vi "Task.vi"() -> (0 "error out":errorcluster)   [LabVIEW 2024]
uses:
  Devices/PCAN/PCAN.lvclass
  ConfigFromJSON/Config from JSON.lvclass
  DBCCommunication/DBC Communication.lvclass
  Devices/HSU MCU V2/HSU MCU V2.lvclass
  Instrument Factory/Instrument Factory.lvclass
  Devices/PCAN/Config Hardcoded/Config Hardcoded.lvclass
  Interfaces/IConfigure/IConfigure.lvclass
  Config from XML/Config from XML.lvclass
panel:
  in  "CAN Adapter Config":T1(ring)
  in  "CAN Adapter":enum16{"PCAN", "X-NET"}(ring)
  out "Temp Winding":dbl
  in  "Stop":bool
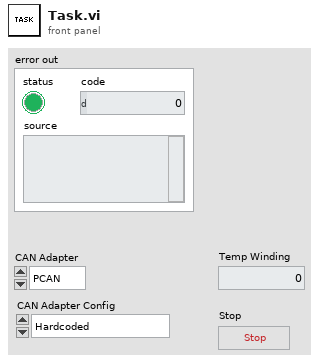
[diagram p1: front panel]
types:
  T1 = enum16{"Hardcoded", "Tests\\PCANconfig.xml", "Tests\\PCANconfig.json"}
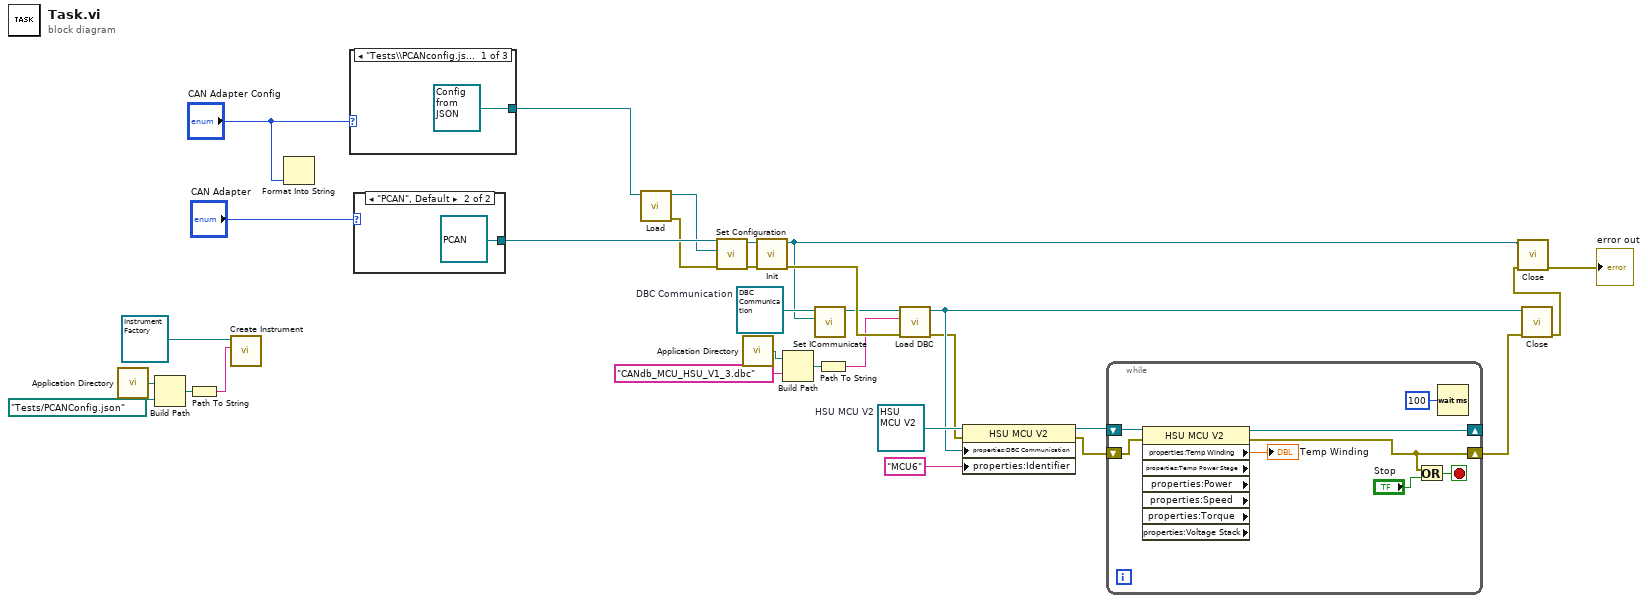
[diagram p0: block diagram]
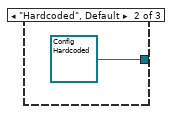
[diagram p3: hidden frame]
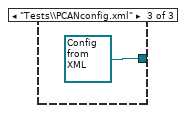
[diagram p4: hidden frame]
diagram:
  w16 = refnum<class "HSU MCU V2.lvclass"> refnum  # HSU MCU V2
  w25 = refnum<class "DBC Communication.lvclass"> refnum  # DBC Communication
  n1 = call <vilib>:"Application Directory.vi"() -> ("Application Directory"=w4:path)
  n2 = Build Path(base path=w4, name or relative path=path "Tests/PCANConfig.json") -> (appended path=w3:path)
  n3 = Path To String(path=w3) -> (string=w1:string)
  n4 = call "Create Instrument.vi"("Source"=w1, "Instrument Factory in"=refnum<class "Instrument Factory.lvclass"> refnum ("Instrument Factory.lvclass")) -> ()  [unwired: 8 in, 2 out]
  n5 = Format Into String("CAN Adapter Config") -> (resulting string=w7:string)  [unwired: 3 in, 1 out]
  n6 = case shown="\"Tests\\\\PCANconfig.json\"" "CAN Adapter Config" {
    tunnel: [refnum<class "Config from JSON.lvclass"> refnum ("Config from JSON.lvclass") refnum<class "Config Hardcoded.lvclass"> refnum ("PCAN.lvlib:Config Hardcoded.lvclass") refnum<class "Config from XML.lvclass"> refnum ("Config from XML.lvclass")] -> w29
    frame "Tests\\PCANconfig.json" {
    }
    frame "Hardcoded", Default {
    }
    frame "Tests\\PCANconfig.xml" {
    }
  }
  n7 = case shown="\"PCAN\", Default" "CAN Adapter" {
    tunnel: [_ refnum<class "PCAN.lvclass"> refnum ("PCAN CAN Adapter")] -> w31
    frame "X-NET" {
    }
    frame "PCAN", Default {
    }
  }
  n8 = call-dynamic "Load.vi"("IConfigure in"=w29) -> ("error out"=w27:errorcluster, "IConfigure out"=w26:refnum<class "IConfigure.lvclass">, "Source"=w17:string)  [unwired: 8 in]
  n9 = call-dynamic "Set Configuration.vi"("IConfigure"=w26, "Copy of PCAN in"=w31) -> ("Copy of PCAN out"=w30:refnum<class "PCAN.lvclass">)  [unwired: 9 in]
  n10 = call <vilib>:"Application Directory.vi"() -> ("Application Directory"=w23:path)
  n11 = call-dynamic "Init.vi"("error in"=w27, "PCAN in"=w30) -> ("error out"=w24:errorcluster, "PCAN out"=w18:refnum<class "PCAN.lvclass">)  [unwired: 8 in]
  n12 = Build Path(base path=w23, name or relative path="CANdb_MCU_HSU_V1_3.dbc" ("Source")) -> (appended path=w21:path)
  n13 = call "Set ICommunicate.vi"("ICommunicate"=w18, "DBCCommunication in"=w25) -> ("DBCCommunication out"=w19:refnum<class "DBC Communication.lvclass">)  [unwired: 9 in]
  n14 = Path To String(path=w21) -> (string=w20:string)
  n15 = call "Load DBC.vi"("error in"=w24, "DBC File"=w20, "DBCCommunication in"=w19) -> ("error out"=w11:errorcluster, "DBCCommunication out"=w12:refnum<class "DBC Communication.lvclass">)  [unwired: 7 in]
  n16 = property class="HSU MCU V2"(reference=w16, error in=w11, "properties:DBC Communication"=w12, "properties:Identifier"="MCU6" ("Instrument Identifier")) -> (reference out=w15:refnum<class "HSU MCU V2.lvclass">, error out=w14:errorcluster)
  n17 = while {
    shift-right: [w36] -> w10
    shift-left: w14 -> [w38]
    shift-right: [w39] -> _
    shift-left: w15 -> [w40]
    stop <- w42 stop-if-true
    n18 = property class="HSU MCU V2" props=["properties:Temp Winding", "properties:Temp Power Stage", "properties:Power", "properties:Speed ", "properties:Torque", "properties:Voltage Stack"](reference=w40, error in=w38) -> (reference out=w39:refnum<class "HSU MCU V2.lvclass">, error out=w36:errorcluster, "properties:Temp Winding"=→"Temp Winding":dbl)  [unwired: 5 out]
    n19 = Or(x=w36, y="Stop") -> (x .or. y?=w42:bool)
    n20 = Wait (ms)(milliseconds to wait=u32 100) -> ()  [unwired: 1 out]
  }
  n21 = call-dynamic "Close.vi"("error in"=w10, "DBC Communication in"=w12) -> ("error out"=w9:errorcluster)  [unwired: 8 in, 1 out]
  n22 = call-dynamic "Close.vi"("error in"=w9, "PCAN in"=w18) -> ("error out"=→"error out":errorcluster)  [unwired: 8 in, 1 out]
